vi "RemoveOpenSet.vi"(9 "Nó":dbl[](array[numeric]), 10 "OpenSet":dbl[][](array[numeric])) -> (2 "NewOpenSet":dbl[][](array[numeric]))   [LabVIEW 2016]
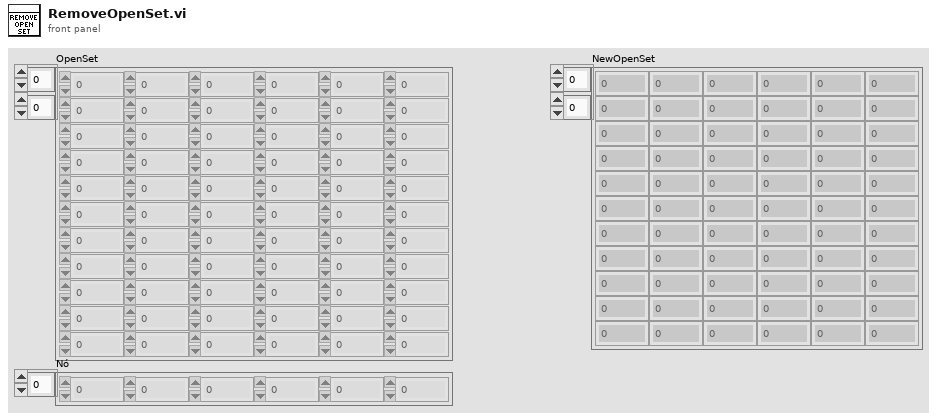
[diagram p1: front panel]
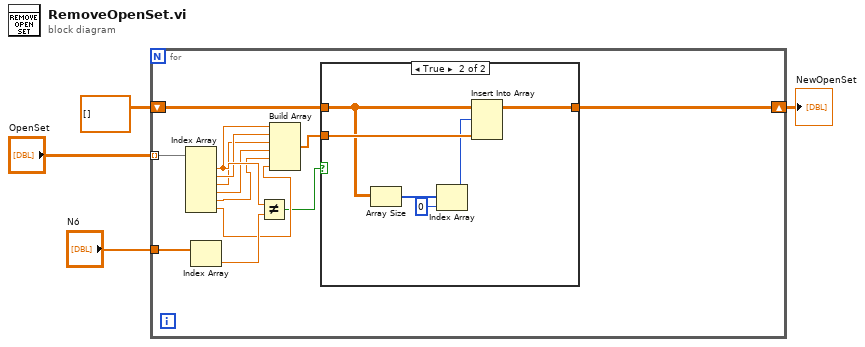
[diagram p0: block diagram]
diagram:
  n1 = for {
    tunnel: "OpenSet" -> [w17] mode=indexing
    tunnel: "Nó" -> [w16]
    shift-right: [w13] -> w1
    shift-left: dbl[][] [] ("Array 2") -> [w14]
    n2 = Index Array(array=w17) -> (element #1=w12:dbl, element #2=w11:dbl, element #3=w10:dbl, element #4=w9:dbl, element #5=w8:dbl, element #6=w7:dbl)  [unwired: 6 in]
    n3 = Index Array(array=w16) -> (element=w15:dbl)  [unwired: 1 in]
    n4 = Not Equal?(x=w12, y=w15) -> (x != y?=w5:bool)
    n5 = Build Array(w12, w11, w10, w9, w8, w7) -> (w6:dbl[])
    n6 = case shown="True" w5 {
      tunnel: w14 -> [w18 w20]
      tunnel: [w18 w24] -> w13
      tunnel: w6 -> [_ w23]
      frame False {
      }
      frame True {
        n7 = Array Size(array=w20) -> (size(s)=w22:i32[])
        n8 = Index Array(array=w22, index=0) -> (element=w19:i32)
        n9 = Insert Into Array(array=w20, index (row)=w19, new element=w23) -> (w24:dbl[][])  [unwired: 1 in]
      }
    }
  }
  "NewOpenSet" <- w1
